vi "Execute.vi"(8 "error in (no error)":errorcluster, 9 "System in":refnum<class "System.lvclass">, 10 "Command in":refnum<class "Command.lvclass">, 11 "State in":refnum<class "State.lvclass">) -> (0 "error out":errorcluster, 2 "Next State":refnum<class "State.lvclass">, 3 "State out":refnum<class "State.lvclass">)   [LabVIEW 2013, in "State.lvclass"]
uses:
  State.lvclass
  Commands/Command/Command.lvclass
  Systems/System/System.lvclass
  State.lvclass/State.ctl
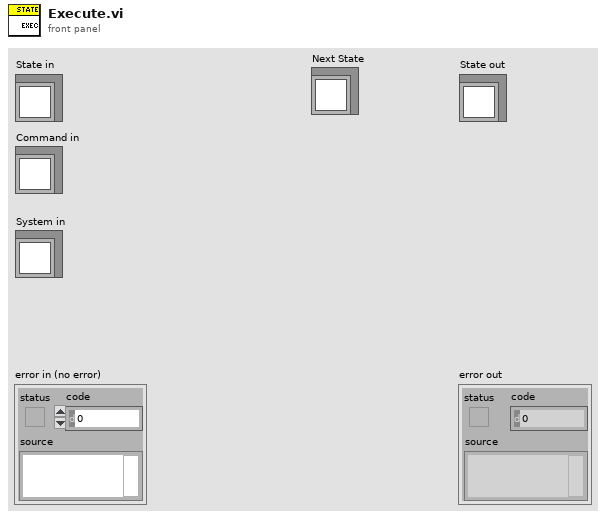
[diagram p1: front panel]
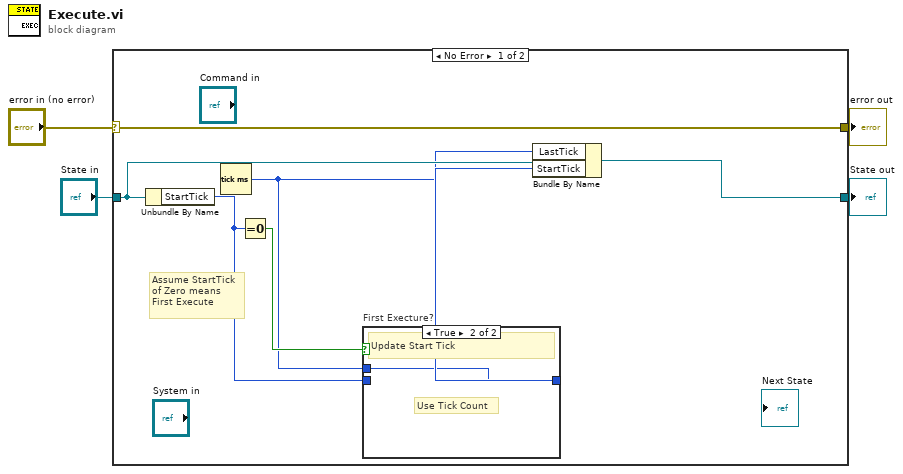
[diagram p0: block diagram]
diagram:
  n1 = case shown="No Error" "error in (no error)" {
    selector: "error in (no error)" -> [w11 w15]
    tunnel: [w11 w15] -> w3
    tunnel: [w10 w14] -> w1
    tunnel: "State in" -> [w9 w14]
    frame No Error {
      # "Assume StartTick\nof Zero means\nFirst Execute"
      n2 = Unbundle By Name(w9) -> ("StartTick"=w6:u32)
      n3 = Tick Count (ms)() -> (millisecond timer value=w5:u32)
      n4 = Equal To 0?(x=w6) -> (x = 0?=w8:bool)
      n5 = case "First Execture?" shown="True" w8 {
        tunnel: [w12 w13] -> w7
        tunnel: w6 -> [w12 _]
        tunnel: w5 -> [_ w13]
        frame False {
          # "Pass Through StartTick"
          # "Not First so don't change start"
        }
        frame True {
          # "Use Tick Count"
          # "Update Start Tick"
        }
      }
      n6 = Bundle By Name(cluster=w9, "LastTick"=w5, "StartTick"=w7) -> (w10:refnum<class "State.lvclass">)
    }
    frame Error {
    }
  }
  "error out" <- w3
  "State out" <- w1
